vi "Flow Low Limit SI.vi"(7 "Set? (F:Read)":bool, 8 "Error In":errorcluster, 9 "Flow Low Limit (0 l/min)":dbl[unit], 10 "Channel (0)":i32, 11 "VISA resource name":refnum<visa-resource-name>) -> (0 "Error Out":errorcluster, 1 "Flow Low Limit out":dbl[unit], 3 "dup VISA resource name":refnum<visa-resource-name>)   [LabVIEW 2012, in "MGC647C.lvlib"]
doc: "Read/Set flow low limit of a channel in SI unit."
uses:
  <instrlib>/MGC647C/MGC647C.lvlib
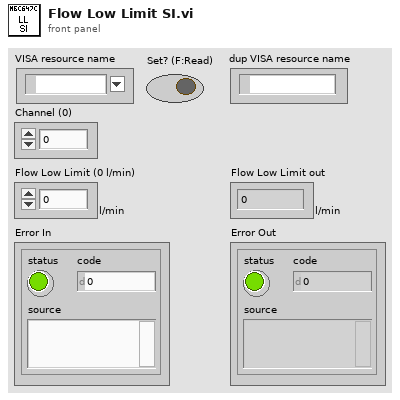
[diagram p1: front panel]
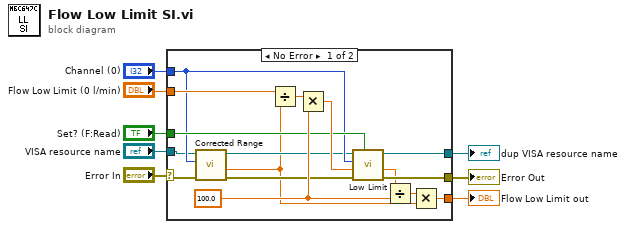
[diagram p0: block diagram]
diagram:
  n1 = case shown="No Error" "Error In" {
    selector: "Error In" -> [w13 w26]
    tunnel: "VISA resource name" -> [w10 w25]
    tunnel: [w24 w25] -> w7
    tunnel: [w23 w26] -> w6
    tunnel: "Set? (F:Read)" -> [w15 _]
    tunnel: "Flow Low Limit (0 l/min)" -> [w19 w27]
    tunnel: [w20 w27] -> w2
    tunnel: "Channel (0)" -> [w14 _]
    frame No Error {
      w17 = 100.0 ("y")
      n2 = call <instrlib>:"Corrected Range.vi"("Error In"=w13, "Channel (0)"=w14, "VISA resource name"=w10) -> ("Error Out"=w12:errorcluster, "Corrected Range"=w9:dbl[unit], "dup VISA resource name"=w11:refnum<visa-resource-name>)  [unwired: 6 in]
      n3 = Divide(x=w19, y=w9) -> (x/y=w18:dbl)
      n4 = Multiply(x=w18, y=w17) -> (x*y=w16:dbl)
      n5 = call <instrlib>:"Low Limit.vi"("Set? (F:Read)"=w15, "Error In"=w12, "Low Limit (0%)"=w16, "Channel (0)"=w14, "VISA resource name"=w11) -> ("Error Out"=w23:errorcluster, "Low Limit out"=w21:dbl, "dup VISA resource name"=w24:refnum<visa-resource-name>)  [unwired: 4 in]
      n6 = Divide(x=w21, y=w17) -> (x/y=w22:dbl)
      n7 = Multiply(x=w22, y=w9) -> (x*y=w20:dbl[unit])
    }
    frame Error {
    }
  }
  "dup VISA resource name" <- w7
  "Error Out" <- w6
  "Flow Low Limit out" <- w2
